vi "Create Evaluations.vi"(8 "error in (no error)":errorcluster, 11 "IEvaluation in":refnum<class "Skyworks_2G_PVT.lvclass">) -> (0 "error out":errorcluster, 2 "Evaluations Out":T1[](array[typedef]) {"Low Limit" format="%#_13g"; "SI Scaling" items=["femto"=-15, "pico"=-12, "nano"=-9, "micro"=-6, "milli"=-3, "percent"=-2, ""=0, "kilo"=3, "mega"=6, "giga"=9, "tera"=12]}, 3 "IEvaluation out":refnum<class "Skyworks_2G_PVT.lvclass">)   [LabVIEW 2016, in "SeqAuto Evaluations.lvlib" / "Skyworks_2G_PVT.lvclass"]
uses:
  Skyworks_2G_PVT.lvclass
  C:/Sequence Automation/Plugins/SeqAuto IEvaluation.lvlibp/SeqAuto IEvaluation.lvclass
  Plugins/TestStand API Tools (TSAT).lvlibp/Evaluation Actions/Includes/Controls/TSAT Evaluation.ctl
  Plugins/TestStand API Tools (TSAT).lvlibp/Evaluation Actions/Includes/Controls/TSAT Eval SI Unit Scaling.ctl
  Plugins/TestStand API Tools (TSAT).lvlibp/Evaluation Actions/Includes/Controls/TSAT Evaluation Type.ctl
  Skyworks_2G_PVT.lvclass/Skyworks_2G_PVT.ctl
  Plugins/SeqAuto IEvaluation.lvlibp/Read Measurement Name.vi
  Plugins/TestStand API Tools (TSAT).lvlibp/Evaluation Actions/TSAT Evaluation Actions.lvlib
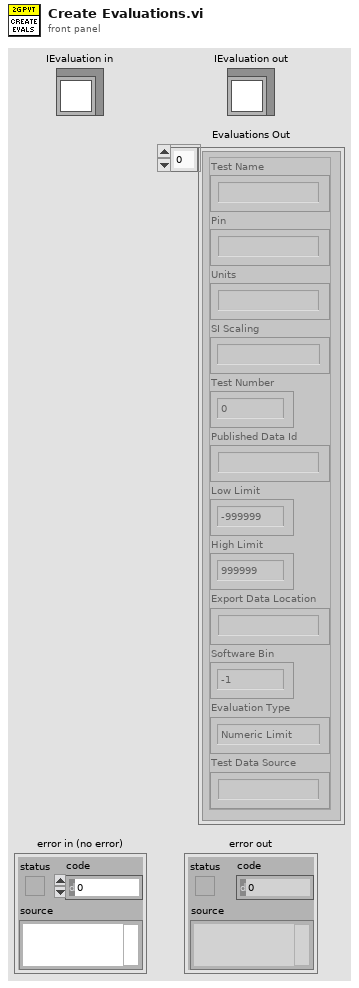
[diagram p1: front panel]
types:
  T1 = typedef "TestStand API Tools (TSAT).lvlibp/TSAT Evaluation Actions.lvlib/TSAT Evaluation.ctl" = cluster{"Test Name":string, "Pin":string, "Units":string, "SI Scaling":T2, "Test Number":i32, "Published Data Id":string, "Low Limit":dbl, "High Limit":dbl, "Export Data Location":string, "Software Bin":i64, "Evaluation Type":T3, "Test Data Source":string}
  T2 = typedef "TestStand API Tools (TSAT).lvlibp/TSAT Evaluation Actions.lvlib/TSAT Eval SI Unit Scaling.ctl" = i16
  T3 = typedef "TestStand API Tools (TSAT).lvlibp/TSAT Evaluation Actions.lvlib/TSAT Evaluation Type.ctl" = enum16{"Numeric Limit", "Pass/Fail", "None"}
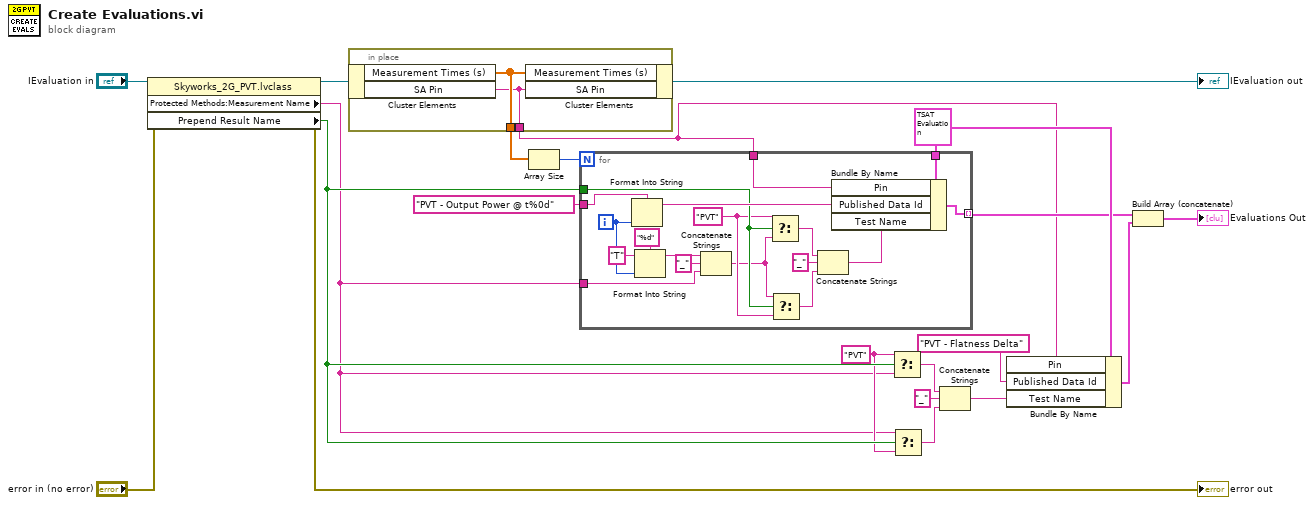
[diagram p0: block diagram]
diagram:
  w9 = "PVT" ("string")
  w15 = T1 {"Test Name"="", "Pin"="", "Units"="", "SI Scaling"=0, "Test Number"=0, "Published Data Id"="", "Low Limit"=-999999.0, "High Limit"=999999.0, "Export Data Location"="", "Software Bin"=-1, "Evaluation Type"=enum."Numeric Limit", "Test Data Source"=""} ("Evaluation")
  n1 = property class="Skyworks_2G_PVT.lvclass"(reference="IEvaluation in", error in="error in (no error)") -> (reference out=w16:refnum<class "Skyworks_2G_PVT.lvclass">, error out=→"error out":errorcluster, "Protected Methods:Measurement Name"=w8:string, "Prepend Result Name"=w10:bool)
  n2 = in-place {
    in-place-border: [w23] -> w19
    in-place-border: [w22] -> w1
    n3 = in-place-cluster #1(w16) -> ("Measurement Times (s)"=w23:dbl[], "SA Pin"=w22:string)
    n4 = in-place-cluster #1("Measurement Times (s)"=w23, "SA Pin"=w22) -> (→"IEvaluation out":refnum<class "Skyworks_2G_PVT.lvclass">)
  }
  n5 = Array Size(array=w19) -> (size(s)=w17:i32)
  n6 = for {
    N: w17 -> [_]
    tunnel: "PVT - Output Power @ t%0d" -> [w24]
    tunnel: w15 -> [w41]
    tunnel: w8 -> [w34]
    tunnel: w10 -> [w32]
    tunnel: [w26] -> w6 mode=indexing
    tunnel: w1 -> [w25]
    i -> [w39]
    w31 = "PVT" ("string")
    n7 = Format Into String(format string=w24, w39) -> (resulting string=w40:string)  [unwired: 2 in, 1 out]
    n8 = Format Into String(format string="%d", initial string="T", w39) -> (resulting string=w36:string)  [unwired: 1 in, 1 out]
    n9 = Concatenate Strings(w36, "_" ("string"), w34) -> (w30:string)
    n10 = Select(t=w31, s=w32, f=w30) -> (s? t:f=w29:string)
    n11 = Select(t=w30, s=w32, f=w31) -> (s? t:f=w28:string)
    n12 = Concatenate Strings(w29, "_" ("string"), w28) -> (w27:string)
    n13 = Bundle By Name(cluster=w41, "Pin"=w25, "Published Data Id"=w40, "Test Name"=w27) -> (w26:T1)
  }
  n14 = Select(t=w9, s=w10, f=w8) -> (s? t:f=w12:string)
  n15 = Select(t=w8, s=w10, f=w9) -> (s? t:f=w11:string)
  n16 = Concatenate Strings(w12, "_" ("string"), w11) -> (w7:string)
  n17 = Bundle By Name(cluster=w15, "Pin"=w1, "Published Data Id"="PVT - Flatness Delta", "Test Name"=w7) -> (w5:T1)
  n18 = Build Array (concatenate)(w6, w5) -> (→"Evaluations Out":T1[])
